vi "Load TestDefinition from XML.vi"(8 "error in (no error)":errorcluster, 11 "TestDefinition":T1={"Test Sequence"=[{"TTrigger"=-130.0, "Direction"=enum."Falling", "TDelay"=0.0, "Type"=enum."No Test", "Pre-Log (s)"=10.0, "Duration (s)"=30.0, "Post-Log(s)"=100.0}, {"TTrigger"=-80.0, "Direction"=enum."Rising", "TDelay"=0.0, "Type"=enum."Heater Test", "Pre-Log (s)"=10.0, "Duration (s)"=30.0, "Post-Log(s)"=100.0}, {"TTrigger"=-50.0, "Direction"=enum."Rising", "TDelay"=30.0, "Type"=enum."Actuation Test", "Pre-Log (s)"=10.0, "Duration (s)"=30.0, "Post-Log(s)"=100.0}, {"TTrigger"=-40.0, "Direction"=enum."Rising", "TDelay"=0.0, "Type"=enum."Actuation Test", "Pre-Log (s)"=10.0, "Duration (s)"=30.0, "Post-Log(s)"=100.0}, {"TTrigger"=-30.0, "Direction"=enum."Rising", "TDelay"=0.0, "Type"=enum."Actuation Test", "Pre-Log (s)"=10.0, "Duration (s)"=30.0, "Post-Log(s)"=100.0}, {"TTrigger"=-20.0, "Direction"=enum."Rising", "TDelay"=0.0, "Type"=enum."Actuation Test", "Pre-Log (s)"=10.0, "Duration (s)"=30.0, "Post-Log(s)"=100.0}, {"TTrigger"=-10.0, "Direction"=enum."Rising", "TDelay"=0.0, "Type"=enum."Actuation Test", "Pre-Log (s)"=10.0, "Duration (s)"=30.0, "Post-Log(s)"=100.0}, {"TTrigger"=0.0, "Direction"=enum."Rising", "TDelay"=0.0, "Type"=enum."Actuation Test", "Pre-Log (s)"=10.0, "Duration (s)"=30.0, "Post-Log(s)"=100.0}, {"TTrigger"=10.0, "Direction"=enum."Rising", "TDelay"=0.0, "Type"=enum."Actuation Test", "Pre-Log (s)"=10.0, "Duration (s)"=30.0, "Post-Log(s)"=100.0}, {"TTrigger"=20.0, "Direction"=enum."Rising", "TDelay"=0.0, "Type"=enum."Actuation Test", "Pre-Log (s)"=10.0, "Duration (s)"=30.0, "Post-Log(s)"=100.0}, {"TTrigger"=30.0, "Direction"=enum."Rising", "TDelay"=0.0, "Type"=enum."Actuation Test", "Pre-Log (s)"=10.0, "Duration (s)"=30.0, "Post-Log(s)"=100.0}, {"TTrigger"=40.0, "Direction"=enum."Rising", "TDelay"=0.0, "Type"=enum."Actuation Test", "Pre-Log (s)"=10.0, "Duration (s)"=30.0, "Post-Log(s)"=100.0}], "ActuationsPerLoop"=10, "Temperature Log Period(ms)"=100, "PSU  Log Period (ms)"=2, "Diode Test Options"={"Temp.Tol"=0.0, "Max IDark"=[], "Min ILight"=[], "Min TEC \nCurrent"=0.0, "Max TEC \nCurrent"=0.0}, "Heater Test Options"={"Heater Nominal Voltage (A)"=0.67, "Heater Voltage Tolerance (%)"=20.0}} {"Heater Test Options"."Heater Voltage Tolerance (%)" min=1.0 max=100.0; "Heater Test Options"."Heater Nominal Voltage (A)" min=0.0 max=1.0; "Test Sequence"."Post-Log(s)" format="%#_13g"; "Test Sequence"."Pre-Log (s)" format="%#_13g"; "Test Sequence"."Duration (s)" format="%#_13g"}) -> (0 "error out":errorcluster, 3 "User Specified Out":T1={"Test Sequence"=[{"TTrigger"=-130.0, "Direction"=enum."Falling", "TDelay"=0.0, "Type"=enum."No Test", "Pre-Log (s)"=10.0, "Duration (s)"=30.0, "Post-Log(s)"=100.0}, {"TTrigger"=-80.0, "Direction"=enum."Rising", "TDelay"=0.0, "Type"=enum."Heater Test", "Pre-Log (s)"=10.0, "Duration (s)"=30.0, "Post-Log(s)"=100.0}, {"TTrigger"=-50.0, "Direction"=enum."Rising", "TDelay"=30.0, "Type"=enum."Actuation Test", "Pre-Log (s)"=10.0, "Duration (s)"=30.0, "Post-Log(s)"=100.0}, {"TTrigger"=-40.0, "Direction"=enum."Rising", "TDelay"=0.0, "Type"=enum."Actuation Test", "Pre-Log (s)"=10.0, "Duration (s)"=30.0, "Post-Log(s)"=100.0}, {"TTrigger"=-30.0, "Direction"=enum."Rising", "TDelay"=0.0, "Type"=enum."Actuation Test", "Pre-Log (s)"=10.0, "Duration (s)"=30.0, "Post-Log(s)"=100.0}, {"TTrigger"=-20.0, "Direction"=enum."Rising", "TDelay"=0.0, "Type"=enum."Actuation Test", "Pre-Log (s)"=10.0, "Duration (s)"=30.0, "Post-Log(s)"=100.0}, {"TTrigger"=-10.0, "Direction"=enum."Rising", "TDelay"=0.0, "Type"=enum."Actuation Test", "Pre-Log (s)"=10.0, "Duration (s)"=30.0, "Post-Log(s)"=100.0}, {"TTrigger"=0.0, "Direction"=enum."Rising", "TDelay"=0.0, "Type"=enum."Actuation Test", "Pre-Log (s)"=10.0, "Duration (s)"=30.0, "Post-Log(s)"=100.0}, {"TTrigger"=10.0, "Direction"=enum."Rising", "TDelay"=0.0, "Type"=enum."Actuation Test", "Pre-Log (s)"=10.0, "Duration (s)"=30.0, "Post-Log(s)"=100.0}, {"TTrigger"=20.0, "Direction"=enum."Rising", "TDelay"=0.0, "Type"=enum."Actuation Test", "Pre-Log (s)"=10.0, "Duration (s)"=30.0, "Post-Log(s)"=100.0}, {"TTrigger"=30.0, "Direction"=enum."Rising", "TDelay"=0.0, "Type"=enum."Actuation Test", "Pre-Log (s)"=10.0, "Duration (s)"=30.0, "Post-Log(s)"=100.0}, {"TTrigger"=40.0, "Direction"=enum."Rising", "TDelay"=0.0, "Type"=enum."Actuation Test", "Pre-Log (s)"=10.0, "Duration (s)"=30.0, "Post-Log(s)"=100.0}], "ActuationsPerLoop"=10, "Temperature Log Period(ms)"=100, "PSU  Log Period (ms)"=2, "Diode Test Options"={"Temp.Tol"=0.0, "Max IDark"=[], "Min ILight"=[], "Min TEC \nCurrent"=0.0, "Max TEC \nCurrent"=0.0}, "Heater Test Options"={"Heater Nominal Voltage (A)"=0.67, "Heater Voltage Tolerance (%)"=20.0}} {"Heater Test Options"."Heater Voltage Tolerance (%)" min=1.0 max=100.0; "Heater Test Options"."Heater Nominal Voltage (A)" min=0.0 max=1.0; "Test Sequence"."Post-Log(s)" format="%#_13g"; "Test Sequence"."Pre-Log (s)" format="%#_13g"; "Test Sequence"."Duration (s)" format="%#_13g"})   [LabVIEW 2025]
doc: "Attempts to load previous user specified settings from an XML file.\n\nThis VI will not generate an error. If a suitable XML file can't be loaded and parsed then it will simply return the default settings."
uses:
  controls/TestDefinition.ctl
  controls/SingleTest.ctl
  controls/TestType.ctl
  controls/Diode Test Options.ctl
  controls/HTR Test Options.ctl
  <vilib>/Utility/xml.llb/Read From XML File(string).vi
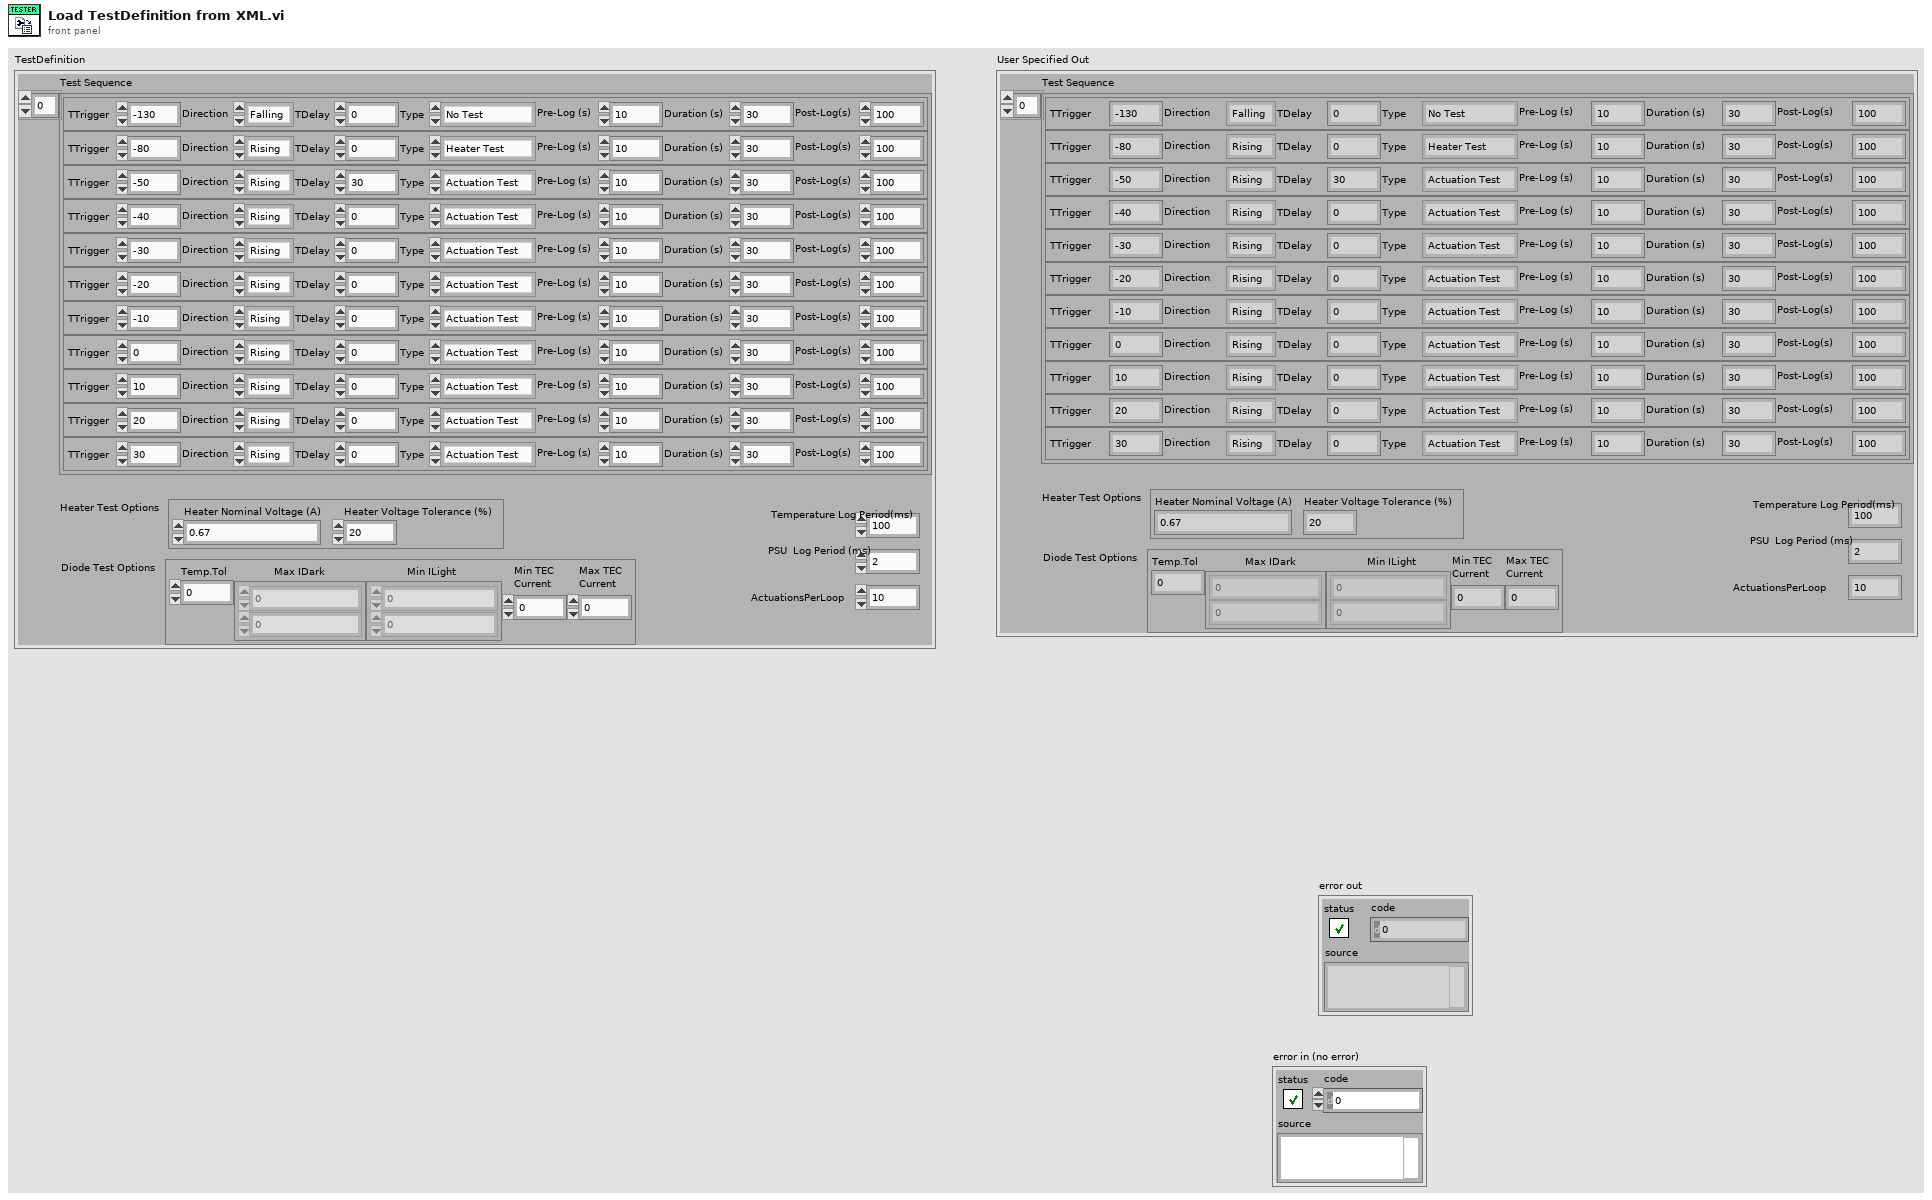
[diagram p1: front panel]
types:
  T1 = typedef "TestDefinition.ctl" = cluster{"Test Sequence":T2[], "ActuationsPerLoop":i32, "Temperature Log Period(ms)":i64, "PSU  Log Period (ms)":i64, "Diode Test Options":T4, "Heater Test Options":T5}
  T2 = typedef "SingleTest.ctl" = cluster{"TTrigger":dbl, "Direction":enum16{"Rising", "Falling"}, "TDelay":dbl, "Type":T3, "Pre-Log (s)":dbl, "Duration (s)":dbl, "Post-Log(s)":dbl}
  T3 = typedef "TestType.ctl" = enum16{"No Test", "Heater Test", "Actuation Test", "Diode Test"}
  T4 = typedef "Diode Test Options.ctl" = cluster{"Temp.Tol":dbl, "Max IDark":dbl[], "Min ILight":dbl[], "Min TEC \nCurrent":dbl, "Max TEC \nCurrent":dbl}
  T5 = typedef "HTR Test Options.ctl" = cluster{"Heater Nominal Voltage (A)":dbl, "Heater Voltage Tolerance (%)":dbl}
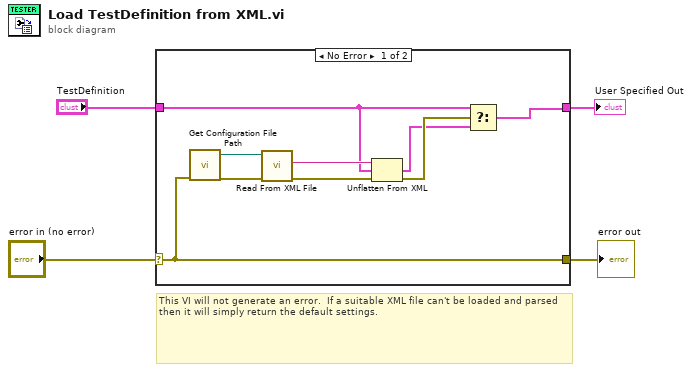
[diagram p0: block diagram]
diagram:
  # "This VI will not generate an error.  If a suitable XML file can't be loaded and parsed then it will simply return the default settings."
  n1 = case shown="No Error" "error in (no error)" {
    selector: "error in (no error)" -> [w10 w15]
    tunnel: [w10 w15] -> w3
    tunnel: "TestDefinition" -> [w7 w14]
    tunnel: [w5 w14] -> w1
    frame No Error {
      n2 = call "Get Configuration File Path.vi"("error in (no error)"=w10) -> ("error out"=w12:errorcluster, "XML File Path"=w13:path)  [unwired: 9 in]
      n3 = call-poly <vilib>:"Read From XML File.vi"("error in (no error)"=w12, "XML File Path"=w13) -> ("error out"=w9:errorcluster, "XML Elements"=w11:string)  [unwired: 7 in, 1 out]
      n4 = Unflatten From XML(xml string=w11, type=w7, error in (no error)=w9) -> (value=w6:T1, error out=w8:errorcluster)
      n5 = Select(t=w7, s=w8, f=w6) -> (s? t:f=w5:T1)
    }
    frame Error {
    }
  }
  "error out" <- w3
  "User Specified Out" <- w1
